vi "Constructor.vi"(8 "error in (no error)":errorcluster, 11 "PlumTomato in":refnum<class "PlumTomato.lvclass">) -> (0 "error out":errorcluster, 2 "Ingredients":string, 3 "PlumTomato out":refnum<class "PlumTomato.lvclass">)   [LabVIEW 2013, in "PlumTomato.lvclass"]
uses:
  PlumTomato.lvclass
panel:
  # "§Ú¬O±ö¤lµf­XÂæ"
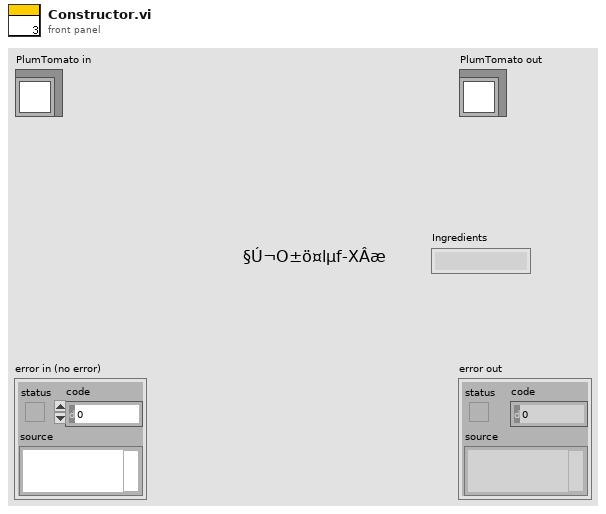
[diagram p1: front panel]
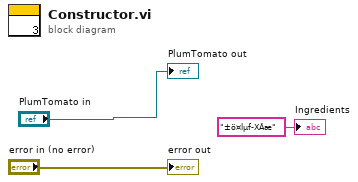
[diagram p0: block diagram]
diagram:
  "error out" <- "error in (no error)"
  "PlumTomato out" <- "PlumTomato in"
  "Ingredients" <- "±ö¤lµf­XÂæ" ("Ingredients")
